vi "IamMouse.vi"() -> ()   [LabVIEW 2013]
uses:
  ObservableQueueData.ctl
  Observable.lvclass/ObserverRegister.ctl
  Mouse.lvclass
  Observable.lvclass/Observable.lvclass
panel:
  in  "UnRegister":bool
  in  "Register":bool
  out "有幾碗飯?":i32
  # "我是Mouse"
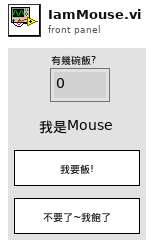
[diagram p1: front panel]
types:
  T1 = typedef "Observable.lvclass/ObserverRegister.ctl" = cluster{"Action":enum16{"Register", "UnRegister"}, "ObserverNotifierReference":refnum<notifier>}
  T2 = typedef "ObservableQueueData.ctl" = cluster{"ObservableAction":enum16{"Null", "Add/RemoveObserver", "NotifyObserver", "GetObserverList"}, "Variant":variant}
  T3 = enum16{"Null", "Add/RemoveObserver", "NotifyObserver"}
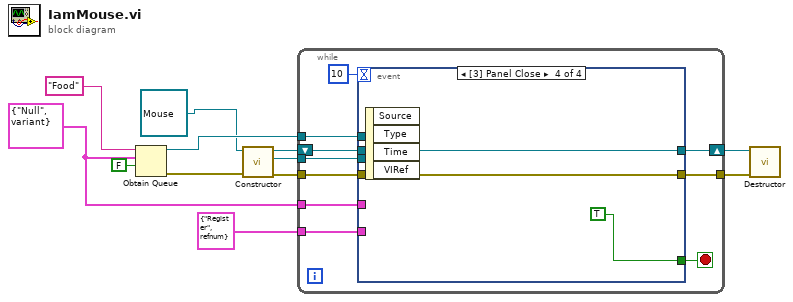
[diagram p0: block diagram]
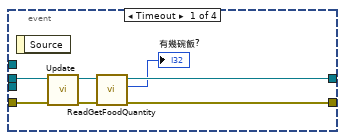
[diagram p2: hidden frame]
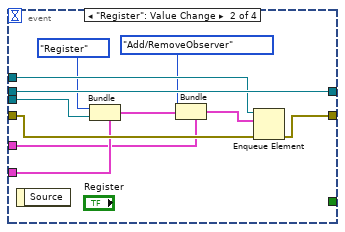
[diagram p3: hidden frame]
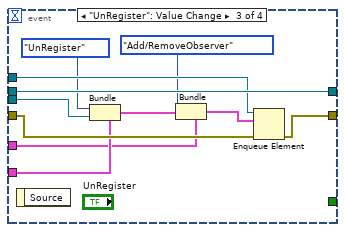
[diagram p4: hidden frame]
diagram:
  w2 = T2 {"ObservableAction"=enum."Null", "Variant"=variant} ("ObservableQueueData")
  n1 = Obtain Queue(name (unnamed)="Food", element data type=w2, create if not found? (T)=FALSE) -> (queue out=w5:refnum<queue>, error out=w6:errorcluster)  [unwired: 2 in, 1 out]
  n2 = call-dynamic "Constructor.vi"("error in (no error)"=w6, "Observer in"=refnum<class "Mouse.lvclass"> refnum ("Mouse.lvclass")) -> ("error out"=w12:errorcluster, "ObserverNotifierReference"=w3:refnum<notifier>, "Observer out"=w9:refnum<class "Mouse.lvclass">)  [unwired: 7 in]
  n3 = while {
    shift-right: [w18] -> w10
    shift-left: w9 -> [w21]
    tunnel: w12 -> [w20]
    tunnel: [w19] -> w11
    tunnel: w5 -> [w16]
    tunnel: T1 {"Action"=enum."Register", "ObserverNotifierReference"=refnum} ("ObserverRegister") -> [w15]
    tunnel: w3 -> [w14]
    tunnel: w2 -> [w13]
    stop <- w17 stop-if-true
    n4 = event shown="[3] Panel Close" {
      selector: _ -> [_ _ _ _]
      dyn-events: _ -> [_ _ _ _]
      timeout: 10 -> [_ _ _ _]
      tunnel: w21 -> [w29 w40 w51 w54]
      tunnel: w20 -> [w28 w38 w49 w53]
      tunnel: [w24 w32 w43 w53] -> w19
      tunnel: [w25 w40 w51 w54] -> w18
      tunnel: [_ _ _ TRUE ("Discard?")] -> w17
      tunnel: w16 -> [_ w39 w50 _]
      tunnel: w15 -> [_ w37 w48 _]
      tunnel: w14 -> [_ w36 w47 _]
      tunnel: w13 -> [_ w35 w46 _]
      event Timeout {
        n5 = event-data() -> ()  [unwired: 1 in, 1 out]
        n6 = call-dynamic "Update.vi"("error in (no error)"=w28, "Duck in"=w29) -> ("error out"=w27:errorcluster, "Duck out"=w26:refnum<class "Mouse.lvclass">)  [unwired: 7 in, 1 out]
        n7 = call-dynamic "ReadGetFoodQuantity.vi"("error in (no error)"=w27, "Duck in"=w26) -> ("error out"=w24:errorcluster, "GetFoodQuantity"=→"有幾碗飯?":i32, "Duck out"=w25:refnum<class "Mouse.lvclass">)  [unwired: 7 in]
      }
      event "Register": Value Change {
        n8 = event-data() -> ()  [unwired: 1 in, 1 out]
        n9 = Bundle(cluster=w37, "Action"=enum16{"Register", "UnRegister"}."Register", "ObserverNotifierReference"=w36) -> (w34:T1)
        n10 = Bundle(cluster=w35, "ObservableAction"=T3."Add/RemoveObserver", "Variant"=w34) -> (w33:T2)
        n11 = Enqueue Element(queue=w39, element=w33, error in (no error)=w38) -> (error out=w32:errorcluster)  [unwired: 1 in, 2 out]
      }
      event "UnRegister": Value Change {
        n12 = event-data() -> ()  [unwired: 1 in, 1 out]
        n13 = Bundle(cluster=w48, "Action"=enum16{"Register", "UnRegister"}."UnRegister", "ObserverNotifierReference"=w47) -> (w45:T1)
        n14 = Bundle(cluster=w46, "ObservableAction"=T3."Add/RemoveObserver", "Variant"=w45) -> (w44:T2)
        n15 = Enqueue Element(queue=w50, element=w44, error in (no error)=w49) -> (error out=w43:errorcluster)  [unwired: 1 in, 2 out]
      }
      event Panel Close {
        n16 = event-data() -> ()  [unwired: 1 in, 4 out]
      }
    }
  }
  n17 = call-dynamic "Destructor.vi"("error in (no error)"=w11, "Observer in"=w10) -> ()  [unwired: 8 in, 2 out]
